vi "ControlShooter.vi"(1 "State":T2) -> (0 "To Shooter\nSolenoid Loop":T1=enum."Forward")   [LabVIEW 2013]
uses:
  typedefs/subStates.ctl
  <vilib>/Rock Robotics/WPI/Solenoid/WPI_SolenoidValue.ctl
  typedefs/fg_typedef.ctl
  <vilib>/Rock Robotics/WPI/Solenoid/WPI_SolenoidGetEnum.vi
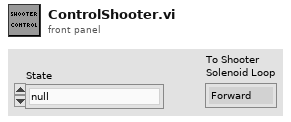
[diagram p1: front panel]
types:
  T1 = typedef "WPI_SolenoidValue.ctl" = enum16{"Off", "On", "Forward", "Reverse"}
  T2 = typedef "subStates.ctl" = enum16{"null", "wait", "driver control", "auto", "manual override", "hold position", "rotate", "pickup", "pass", "load", "goto shoot", "shoot", "end"}
  T3 = typedef "fg_typedef.ctl" = enum16{"Get", "Set"}
  T4 = typedef "WPI_DigitalInputDevRef.ctl" = cluster{"DevStatus":errorcluster, "DIO Channel":T5, "Digital Module":T6}
  T5 = typedef "FPGA_DIOChannel.ctl" = enum8{"DIO 1", "DIO 2", "DIO 3", "DIO 4", "DIO 5", "DIO 6", "DIO 7", "DIO 8", "DIO 9", "DIO 10", "DIO 11", "DIO 12", "DIO 13", "DIO 14", "Invalid"}
  T6 = typedef "FPGA_TypedefDigitalModule.ctl" = enum16{"Digital Module 1", "Digital Module 2"}
  T7 = typedef "WPI_SolenoidDevRef.ctl" = cluster{"DevStatus":errorcluster, "Solenoid Module":T8, "Forward Solenoid Channel":T9, "Reverse Solenoid Channel":T9}
  T8 = typedef "FPGA_TypedefSolenoidModule.ctl" = enum16{"Solenoid Module 1", "Solenoid Module 2"}
  T9 = typedef "WPI_SolenoidChannel.ctl" = enum8{"Solenoid 1", "Solenoid 2", "Solenoid 3", "Solenoid 4", "Solenoid 5", "Solenoid 6", "Solenoid 7", "Solenoid 8", "Invalid"}
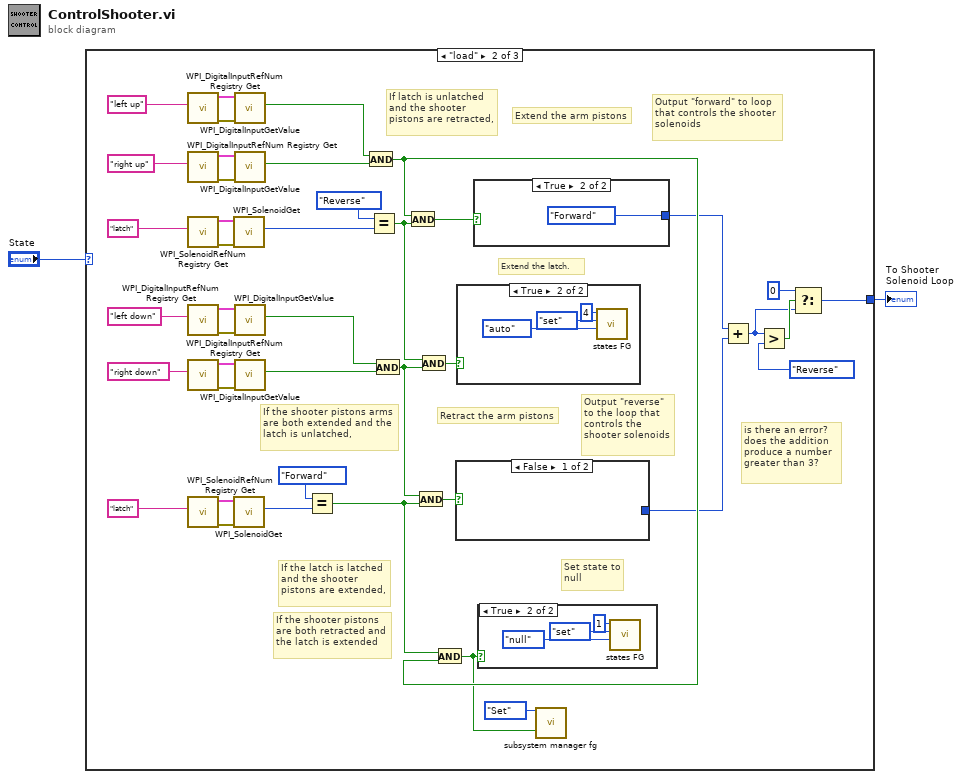
[diagram p0: block diagram]
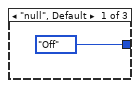
[diagram p2: hidden frame]
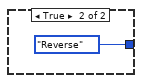
[diagram p4: hidden frame]
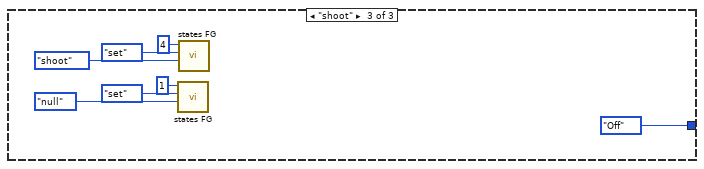
[diagram p7: hidden frame]
diagram:
  n1 = case shown="\"load\"" "State" {
    tunnel: [WPI_SolenoidValue."Off" ("To Shooter\nSolenoid Loop") w7 WPI_SolenoidValue."Off" ("To Shooter\nSolenoid Loop")] -> w1
    frame "null", Default {
    }
    frame "load" {
      # "is there an error?\ndoes the addition\nproduce a number \ngreater than 3?"
      # "Output \"reverse\"\nto the loop that\ncontrols the\nshooter solenoids"
      # "Output \"forward\" to loop\nthat controls the shooter\nsolenoids"
      # "Set state to\nnull"
      # "If the shooter pistons\nare both retracted and\nthe latch is extended"
      # "If the latch is latched\nand the shooter\npistons are extended,"
      # "Retract the arm pistons"
      # "If latch is unlatched\nand the shooter\npistons are retracted,"
      # "Extend the latch."
      # "If the shooter pistons arms\nare both extended and the\nlatch is unlatched,"
      # "Extend the arm pistons"
      n2 = call <vilib>:"WPI_DigitalInputRefNum Registry Get.vi"("refnum name"="left up") -> ("error out"=w36:errorcluster, "DigitalInputDevRef"=w37:T4)  [unwired: 9 in]
      n3 = call <vilib>:"WPI_DigitalInputRefNum Registry Get.vi"("refnum name"="right up") -> ("error out"=w39:errorcluster, "DigitalInputDevRef"=w40:T4)  [unwired: 9 in]
      n4 = call <vilib>:"WPI_SolenoidRefNum Registry Get.vi"("refnum name"="latch") -> ("error out"=w45:errorcluster, "SolenoidDevRef"=w44:T7)  [unwired: 9 in]
      n5 = call <vilib>:"WPI_DigitalInputRefNum Registry Get.vi"("refnum name"="left down") -> ("error out"=w29:errorcluster, "DigitalInputDevRef"=w30:T4)  [unwired: 9 in]
      n6 = call <vilib>:"WPI_DigitalInputRefNum Registry Get.vi"("refnum name"="right down") -> ("error out"=w26:errorcluster, "DigitalInputDevRef"=w27:T4)  [unwired: 9 in]
      n7 = call <vilib>:"WPI_SolenoidRefNum Registry Get.vi"("refnum name"="latch") -> ("error out"=w22:errorcluster, "SolenoidDevRef"=w21:T7)  [unwired: 9 in]
      n8 = call-poly <vilib>:"WPI_SolenoidGet.vi"("error in (no error)"=w45, "SolenoidDevRef"=w44) -> ("Value"=w42:T1)  [unwired: 7 in, 2 out]
      n9 = call-poly <vilib>:"WPI_SolenoidGet.vi"("error in (no error)"=w22, "SolenoidDevRef"=w21) -> ("Value"=w19:T1)  [unwired: 7 in, 2 out]
      n10 = call <vilib>:"WPI_DigitalInputGetValue.vi"("error in (no error)"=w36, "DigitalInputDevRef"=w37) -> ("Value"=w34:bool)  [unwired: 7 in, 2 out]
      n11 = call <vilib>:"WPI_DigitalInputGetValue.vi"("error in (no error)"=w39, "DigitalInputDevRef"=w40) -> ("Value"=w33:bool)  [unwired: 7 in, 2 out]
      n12 = call <vilib>:"WPI_DigitalInputGetValue.vi"("error in (no error)"=w29, "DigitalInputDevRef"=w30) -> ("Value"=w24:bool)  [unwired: 7 in, 2 out]
      n13 = call <vilib>:"WPI_DigitalInputGetValue.vi"("error in (no error)"=w26, "DigitalInputDevRef"=w27) -> ("Value"=w23:bool)  [unwired: 7 in, 2 out]
      n14 = Equal?(x=WPI_SolenoidValue."Forward", y=w19) -> (x = y?=w14:bool)
      n15 = And(x=w34, y=w33) -> (x .and. y?=w13:bool)
      n16 = Equal?(x=WPI_SolenoidValue."Reverse", y=w42) -> (x = y?=w15:bool)
      n17 = And(x=w24, y=w23) -> (x .and. y?=w16:bool)
      n18 = And(x=w13, y=w15) -> (x .and. y?=w32:bool)
      n19 = And(x=w16, y=w14) -> (x .and. y?=w17:bool)
      n20 = And(x=w15, y=w16) -> (x .and. y?=w31:bool)
      n21 = And(x=w14, y=w13) -> (x .and. y?=w4:bool)
      n22 = case shown="False" w17 {
        tunnel: [_ WPI_SolenoidValue."Reverse" ("Value")] -> w6
        frame False {
        }
        frame True {
        }
      }
      n23 = case shown="True" w31 {
        frame False {
        }
        frame True {
          n24 = call "states FG.vi"("subState in"=subStates."auto", "menu (get)"=enum16{"set", "get"}."set", "Loop ID"=4) -> ()  [unwired: 5 in, 4 out]
        }
      }
      n25 = case shown="True" w32 {
        tunnel: [_ WPI_SolenoidValue."Forward" ("Value")] -> w12
        frame False {
        }
        frame True {
        }
      }
      n26 = case shown="True" w4 {
        frame False {
        }
        frame True {
          n27 = call "states FG.vi"("subState in"=subStates."null", "menu (get)"=enum16{"set", "get"}."set", "Loop ID"=1) -> ()  [unwired: 5 in, 4 out]
        }
      }
      n28 = call "subsystem manager fg.vi"("Menu"=fg_typedef."Set", "Shooter Cocked"=w4) -> ()  [unwired: 13 in, 5 out]
      n29 = Add(x=w12, y=w6) -> (x+y=w9:u16)
      n30 = Greater?(x=w9, y=WPI_SolenoidValue."Reverse" ("Value")) -> (0:w10:bool)
      n31 = Select(t=0, s=w10, f=w9) -> (s? t:f=w7:i32)
    }
    frame "shoot" {
      n32 = call "states FG.vi"("subState in"=subStates."null", "menu (get)"=enum16{"set", "get"}."set", "Loop ID"=1) -> ()  [unwired: 5 in, 4 out]
      n33 = call "states FG.vi"("subState in"=subStates."shoot", "menu (get)"=enum16{"set", "get"}."set", "Loop ID"=4) -> ()  [unwired: 5 in, 4 out]
    }
  }
  "To Shooter\nSolenoid Loop" <- w1
